vi "Variant_InsertElementIntoCluster.vi"(7 "insert index (-1: end)":i32=-1, 9 "Element Name":string, 10 "Element":variant, 11 "Cluster in":variant) -> (3 "Cluster out":variant)   [LabVIEW 2020, in "OpenVariant.lvlib"]
uses:
  OpenVariant.lvlib
  _built_ppls/OpenDescriptor.lvlibp
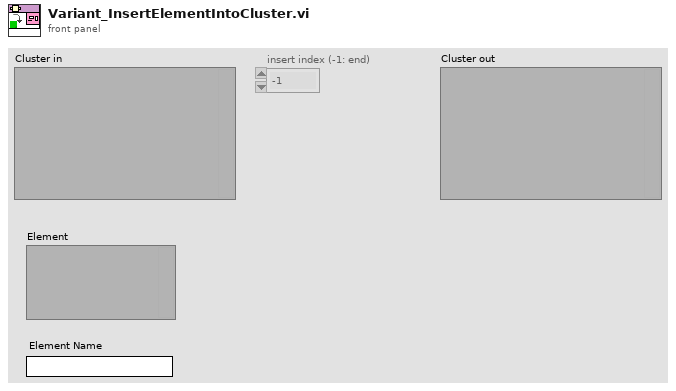
[diagram p1: front panel]
types:
  T1 = typedef "OpenDescriptor.lvlibp/OpenDescriptor -- cluster.ctl" = cluster{"type descriptor":i16[], "name":string, "class":string, "data string":string}
  T2 = typedef "Type Descriptor I16 Array.ctl" = T3[]
  T3 = typedef "Type Descriptor I16.ctl" = i16
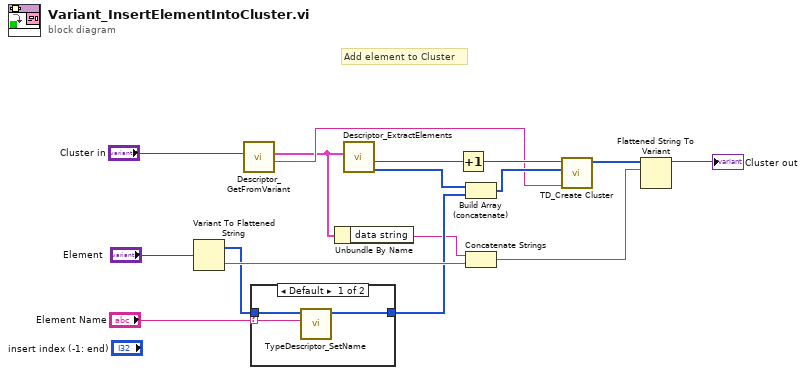
[diagram p0: block diagram]
diagram:
  # "Add element to Cluster"
  n1 = Variant To Flattened String(Variant="Element") -> (data string=w13:string, 1:w10:i16[])
  n2 = call "Descriptor_GetFromVariant.vi"("Variant"="Cluster in") -> ("name"=w4:string, "Descriptor"=w3:T1)  [unwired: 9 in]
  n3 = case shown="Default" "Element Name" {
    selector: "Element Name" -> [w17 _]
    tunnel: w10 -> [w19 w20]
    tunnel: [w18 w20] -> w9
    frame Default {
      n4 = call "TypeDescriptor_SetName.vi"("name"=w17, "type descriptor"=w19) -> ("type descriptor dup"=w18:i16[])  [unwired: 7 in, 2 out]
    }
    frame "" {
    }
  }
  n5 = Unbundle By Name(w3) -> ("data string"=w6:string)
  n6 = call "Descriptor_ExtractElements.vi"("Descriptor"=w3) -> ("concatenated element descriptors"=w1:i16[], "Nb elements"=w2:i32)  [unwired: 8 in, 1 out]
  n7 = Increment(x=w2) -> (x+1=w8:i32)
  n8 = Build Array (concatenate)(w1, w9) -> (w16:i16[])
  n9 = Concatenate Strings(w6, w13) -> (w14:string)
  n10 = call <vilib>:"TD_Create Cluster.vi"("Name"=w4, "Concatenated Elts"=w16, "N Elts"=w8) -> ("ClusterTD"=w15:T2)  [unwired: 8 in]
  n11 = Flattened String To Variant(6:w14, 7:w15) -> (3:→"Cluster out":variant)  [unwired: 1 in, 1 out]
